vi "Acquire GPS_Heading.vi"(11 "GPS COM Port":refnum<visa-resource-name>) -> (3 "Lat, long, heading output":dbl[](array[numeric]))   [LabVIEW 2014]
panel:
  # "Acquire GPS with Heading"
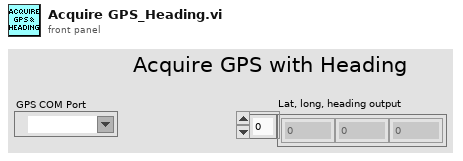
[diagram p1: front panel]
types:
  T1 = cluster{"UTC Time":timestamp, "Local Time":timestamp, "Lattitude (ddmm.mmmm)":dbl, "Lattitude North/South":string, "Longitude (ddmm.mmmm)":dbl, "Longitude East/West":string, "Magnetic Variation (degrees)":dbl, "Variation East/West":string, "Speed over ground (knots)":dbl, "Course over ground (degrees)":dbl}
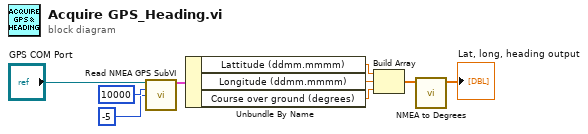
[diagram p0: block diagram]
diagram:
  n1 = call "Read NMEA GPS SubVI.vi"("VISA resource name"="GPS COM Port", "timeout (ms)"=10000, "UTC Time Zone"=-5) -> ("GPS Data"=w6:T1)  [unwired: 9 in, 3 out]
  n2 = Unbundle By Name(w6) -> ("Lattitude (ddmm.mmmm)"=w5:dbl, "Longitude (ddmm.mmmm)"=w4:dbl, "Course over ground (degrees)"=w3:dbl)
  n3 = Build Array(w5, w4, w3) -> (w2:dbl[])
  n4 = call "NMEA to Degrees.vi"("NMEA Input"=w2) -> ("Degrees Output"=→"Lat, long, heading output":dbl[])  [unwired: 10 in]
